vi "ma_SML RT Zoom FFT Settings.vi"(6 "effective band specification":cluster{"fl":dbl, "fh":dbl}={"fl"=0.0, "fh"=0.5} {"fh" format="%.2f"; "fl" format="%.2f"}, 7 "RBW definition":enum16{"3dB", "6dB", "ENBW", "bin width"}(ring), 8 "error in (no error)":errorcluster, 9 "input signal type":enum16{"real", "complex modulated"}(ring), 10 "fs":dbl=1024.0 format="%.2f", 11 "spectrum settings":T1={"center frequency"=-inf, "span"=-1.0, "resolution bandwidth"=-1.0, "window"=0, "spectral lines"=-1, "%overlap"=0.0} {"%overlap" min=0.0 max=100.0 format="%.2f"; "window" items=["Rectangle"=0, "Hanning"=1, "Hamming"=2, "Blackman-Harris"=3, "Exact Blackman"=4, "Blackman"=5, "Flat Top"=6, "4 Term B-Harris "=7, "7 Term B-Harris"=8, "Low Sidelobe"=9, "Blackman Nuttall"=11, "Triangle"=30, "Bartlett-Hanning"=31, "Bohman"=32, "Parzen"=33, "Welch"=34, "Kaiser"=60, "Dolph-Chebyshev"=61, "Gaussian"=62]; "resolution bandwidth" format="%.2p"; "center frequency" format="%.2p"; "span" format="%.2p"}) -> (0 "error out":errorcluster, 2 "zoom FFT settings":T2={"zoom settings"={"center frequency"=-inf, "zoom"=1, "trim"=1.0}, "FFT settings"={"window"=1, "window size"=1024, "FFT size"=-1, "%overlap"=0.0}} {"FFT settings"."%overlap" min=0.0 max=100.0 format="%.2f"; "FFT settings"."window" items=["Rectangle"=0, "Hanning"=1, "Hamming"=2, "Blackman-Harris"=3, "Exact Blackman"=4, "Blackman"=5, "Flat Top"=6, "4 Term B-Harris "=7, "7 Term B-Harris"=8, "Low Sidelobe"=9, "Blackman Nuttall"=11, "Triangle"=30, "Bartlett-Hanning"=31, "Bohman"=32, "Parzen"=33, "Welch"=34, "Kaiser"=60, "Dolph-Chebyshev"=61, "Gaussian"=62]; "zoom settings"."trim" min=1.0 format="%.2f"; "zoom settings"."center frequency" format="%.2f"; "zoom settings"."zoom" min=1}, 3 "actual spectrum settings":T1={"center frequency"=-inf, "span"=-1.0, "resolution bandwidth"=-1.0, "window"=0, "spectral lines"=-1, "%overlap"=0.0} {"%overlap" min=0.0 max=100.0 format="%.2f"; "window" items=["Rectangle"=0, "Hanning"=1, "Hamming"=2, "Blackman-Harris"=3, "Exact Blackman"=4, "Blackman"=5, "Flat Top"=6, "4 Term B-Harris "=7, "7 Term B-Harris"=8, "Low Sidelobe"=9, "Blackman Nuttall"=11, "Triangle"=30, "Bartlett-Hanning"=31, "Bohman"=32, "Parzen"=33, "Welch"=34, "Kaiser"=60, "Dolph-Chebyshev"=61, "Gaussian"=62]; "resolution bandwidth" format="%.2p"; "center frequency" format="%.2p"; "span" format="%.2p"}, 5 "max block size":i32)   [LabVIEW 2020, in "NI_MAPro.lvlib"]
uses:
  NI_MAPro.lvlib
  ma_sml_CZ Spectrum Settings.ctl
  ma_sml_RT Zoom FFT Settings.ctl
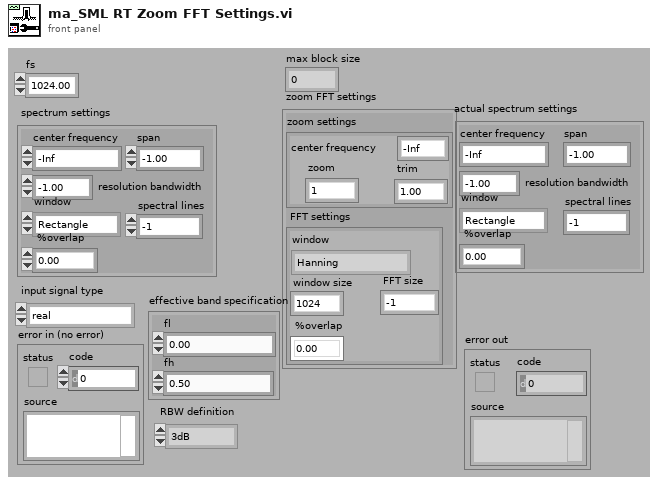
[diagram p1: front panel]
types:
  T1 = typedef "NI_MAPro.lvlib/ma_sml_CZ Spectrum Settings.ctl" = cluster{"center frequency":dbl, "span":dbl, "resolution bandwidth":dbl, "window":u16, "spectral lines":i32, "%overlap":dbl}
  T2 = typedef "NI_MAPro.lvlib/ma_sml_RT Zoom FFT Settings.ctl" = cluster{"zoom settings":cluster{"center frequency":dbl, "zoom":i32, "trim":dbl}, "FFT settings":cluster{"window":u16, "window size":i32, "FFT size":i32, "%overlap":dbl}}
  T3 = cluster{"actual RBW":dbl, "max block size":i32, "settings":T2}
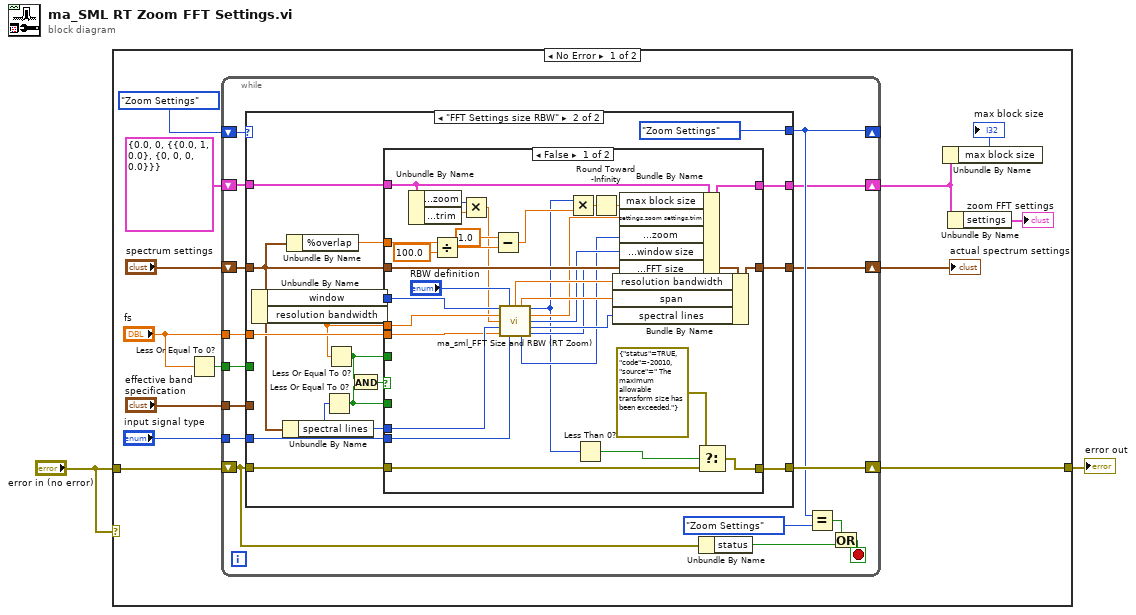
[diagram p0: block diagram]
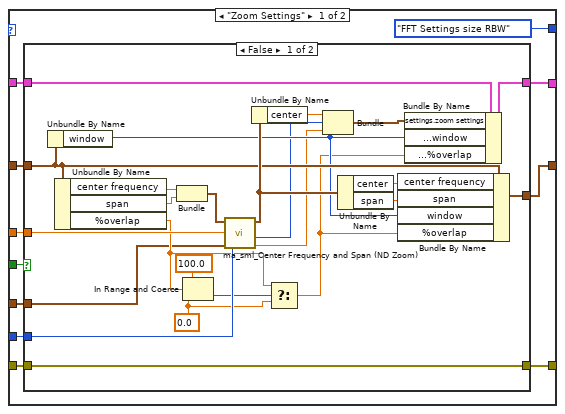
[diagram p2: hidden frame]
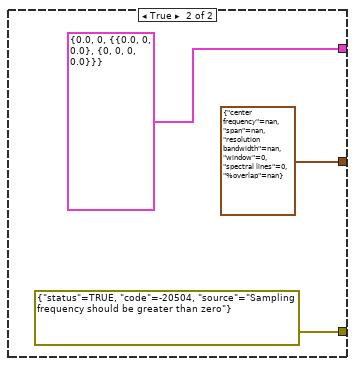
[diagram p3: hidden frame]
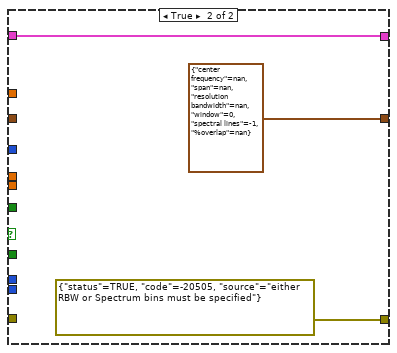
[diagram p4: hidden frame]
diagram:
  n1 = case shown="No Error" "error in (no error)" {
    tunnel: "error in (no error)" -> [w15 w121]
    tunnel: [w14 w121] -> w2
    frame No Error {
      n2 = Less Or Equal To 0?(x="fs") -> (x <= 0?=w7:bool)
      n3 = while {
        tunnel: "effective band specification" -> [w16]
        tunnel: "input signal type" -> [w17]
        tunnel: w7 -> [w18]
        shift-left: "spectrum settings" -> [w21]
        shift-right: [w20] -> w10
        shift-left: w15 -> [w25]
        shift-right: [w24] -> w14
        shift-left: enum16{"Zoom Settings", "FFT Settings size RBW"}."Zoom Settings" -> [w29]
        shift-right: [w23] -> _
        shift-left: T3 {"actual RBW"=0.0, "max block size"=0, "settings"={"zoom settings"={"center frequency"=0.0, "zoom"=1, "trim"=0.0}, "FFT settings"={"window"=0, "window size"=0, "FFT size"=0, "%overlap"=0.0}}} -> [w30]
        shift-right: [w22] -> w13
        tunnel: "fs" -> [w31]
        stop <- w26 stop-if-true
        n4 = case shown="\"FFT Settings size RBW\"" w29 {
          tunnel: w31 -> [w37 w79]
          tunnel: w30 -> [w35 w76]
          tunnel: [w34 w75] -> w22
          tunnel: w25 -> [w39 w82]
          tunnel: [w40 w81] -> w24
          tunnel: [enum16{"Zoom Settings", "FFT Settings size RBW"}."FFT Settings size RBW" enum16{"Zoom Settings", "FFT Settings size RBW"}."Zoom Settings"] -> w23
          tunnel: w21 -> [w38 w71]
          tunnel: [w36 w72] -> w20
          tunnel: w18 -> [w41 _]
          tunnel: w17 -> [w33 w73]
          tunnel: w16 -> [w32 _]
          frame "Zoom Settings" {
            n5 = case shown="False" w41 {
              tunnel: w39 -> [w66 _]
              tunnel: [w66 errorcluster {"status"=TRUE, "code"=-20504, "source"="Sampling frequency should be greater than zero"} ("error in (no error)")] -> w40
              tunnel: w38 -> [w52 _]
              tunnel: w37 -> [w64 _]
              tunnel: [w65 T1 {"center frequency"=nan, "span"=nan, "resolution bandwidth"=nan, "window"=0, "spectral lines"=0, "%overlap"=nan} ("spectrum settings")] -> w36
              tunnel: [w56 T3 {"actual RBW"=0.0, "max block size"=0, "settings"={"zoom settings"={"center frequency"=0.0, "zoom"=0, "trim"=0.0}, "FFT settings"={"window"=0, "window size"=0, "FFT size"=0, "%overlap"=0.0}}}] -> w34
              tunnel: w35 -> [w57 _]
              tunnel: w33 -> [w60 _]
              tunnel: w32 -> [w45 _]
              frame False {
                w47 = 0.0 ("lower limit")
                n6 = Unbundle By Name(w52) -> ("window"=w51:u16)
                n7 = Unbundle By Name(w52) -> ("center frequency"=w63:dbl, "span"=w62:dbl, "%overlap"=w48:dbl)
                n8 = Bundle("center frequency"=w63, "span"=w62) -> (w61:cluster{"center frequency":dbl, "span":dbl})  [unwired: 1 out]
                n9 = In Range and Coerce(upper limit=100.0, x=w48, lower limit=w47) -> (In Range?=w49:bool)  [unwired: 1 out]
                n10 = call "ma_sml_Center Frequency and Span (ND Zoom).vi"("effective band specification"=w45, "input signal type"=w60, "fs"=w64, "desired center span"=w61) -> ("trim"=w43:dbl, "zoom"=w44:i32, "actual center span"=w55:cluster{"center":dbl, "span":dbl})  [unwired: 1 out]
                n11 = Unbundle By Name(w55) -> ("center"=w54:dbl)
                n12 = Select(t=w48, s=w49, f=w47) -> (s? t:f=w46:dbl)
                n13 = Bundle("center"=w54, "zoom"=w44, "trim"=w43) -> (w53:cluster{"center":dbl, "zoom":i32, "trim":dbl})  [unwired: 1 out]
                n14 = Unbundle By Name(w55) -> ("center"=w59:dbl, "span"=w58:dbl)
                n15 = Bundle By Name(cluster=w52, "center frequency"=w59, "span"=w58, "window"=w51, "%overlap"=w46) -> (w65:T1)
                n16 = Bundle By Name(cluster=w57, "settings.zoom settings"=w53, "settings.FFT settings.window"=w51, "settings.FFT settings.%overlap"=w46) -> (w56:T3)
              }
              frame True {
              }
            }
          }
          frame "FFT Settings size RBW" {
            n17 = Unbundle By Name(w71) -> ("window"=w80:u16, "resolution bandwidth"=w78:dbl)
            n18 = Unbundle By Name(w71) -> ("spectral lines"=w85:i32)
            n19 = Unbundle By Name(w71) -> ("%overlap"=w70:dbl)
            n20 = Less Or Equal To 0?(x=w85) -> (x <= 0?=w77:bool)
            n21 = Less Or Equal To 0?(x=w78) -> (x <= 0?=w84:bool)
            n22 = And(x=w84, y=w77) -> (x .and. y?=w83:bool)
            n23 = case shown="False" w83 {
              tunnel: w82 -> [w88 _]
              tunnel: [w87 errorcluster {"status"=TRUE, "code"=-20505, "source"="either RBW or Spectrum bins must be specified"} ("error in (no error)")] -> w81
              tunnel: w84 -> [_ _]
              tunnel: w80 -> [w117 _]
              tunnel: w79 -> [w114 _]
              tunnel: w78 -> [w116 _]
              tunnel: w77 -> [_ _]
              tunnel: w76 -> [w106 w119]
              tunnel: w85 -> [w115 _]
              tunnel: [w107 w119] -> w75
              tunnel: [w112 T1 {"center frequency"=nan, "span"=nan, "resolution bandwidth"=nan, "window"=0, "spectral lines"=-1, "%overlap"=nan} ("spectrum settings")] -> w72
              tunnel: w71 -> [w111 _]
              tunnel: w73 -> [w113 _]
              tunnel: w70 -> [w102 _]
              frame False {
                n24 = Unbundle By Name(w106) -> ("settings.zoom settings.zoom"=w93:i32, "settings.zoom settings.trim"=w92:dbl)
                n25 = Divide(x=w102, y=100.0) -> (x/y=w99:dbl)
                n26 = Multiply(x=w93, y=w92) -> (x*y=w94:dbl)
                n27 = Subtract(x=1.0, y=w99) -> (x-y=w97:dbl)
                n28 = call "ma_sml_FFT Size and RBW (RT Zoom).vi"("window"=w117, "RBW definition"="RBW definition", "RBW"=w116, "zoom"=w94, "spectral lines"=w115, "fs"=w114, "input signal type"=w113) -> ("RBW actual"=w110:dbl, "span"=w109:dbl, "block size"=w90:i32, "trim"=w105:dbl, "window size"=w103:i32, "spectral lines actual"=w108:i32, "zoom factor"=w91:i32, "FFT Size"=w104:i32)  [unwired: 1 out]
                n29 = Multiply(x=w90, y=w97) -> (x*y=w100:dbl)
                n30 = Less Than 0?(x=w90) -> (x < 0?=w89:bool)
                n31 = Round Toward -Infinity(1:w100) -> (0:w98:dbl)
                n32 = Bundle By Name(cluster=w111, "resolution bandwidth"=w110, "span"=w109, "spectral lines"=w108) -> (w112:T1)
                n33 = Bundle By Name(cluster=w106, "max block size"=w98, "settings.zoom settings.trim"=w105, "settings.zoom settings.zoom"=w91, "settings.FFT settings.window size"=w103, "settings.FFT settings.FFT size"=w104) -> (w107:T3)
                n34 = Select(t=errorcluster {"status"=TRUE, "code"=-20010, "source"=" The maximum allowable transform size has been exceeded."}, s=w89, f=w88) -> (s? t:f=w87:errorcluster)
              }
              frame True {
              }
            }
          }
        }
        n35 = Unbundle By Name(w25) -> ("status"=w27:bool)
        n36 = Equal?(x=w23, y=enum16{"Zoom Settings", "FFT Settings size RBW"}."Zoom Settings") -> (x = y?=w28:bool)
        n37 = Or(x=w28, y=w27) -> (x .or. y?=w26:bool)
      }
      "actual spectrum settings" <- w10
      n38 = Unbundle By Name(w13) -> ("max block size"=→"max block size":i32)
      n39 = Unbundle By Name(w13) -> ("settings"=→"zoom FFT settings":T2)
    }
    frame Error {
    }
  }
  "error out" <- w2
